vi "Apply_RF.vi"(0 "I- index":dbl, 4 "I+ index":dbl, 5 "RF Proportional to intensity":bool, 6 "RF Target Position":i32, 7 "RF indicator":bool, 8 "RF Power":dbl, 9 "rho0":dbl[](array[numeric]), 10 "rho-":dbl[](array[numeric]), 11 "rho+":dbl[](array[numeric])) -> (1 "rho- out":dbl[](array[numeric]), 2 "rho0 out":dbl[](array[numeric]), 3 "rho+ out":dbl[](array[numeric]))   [LabVIEW 2018]
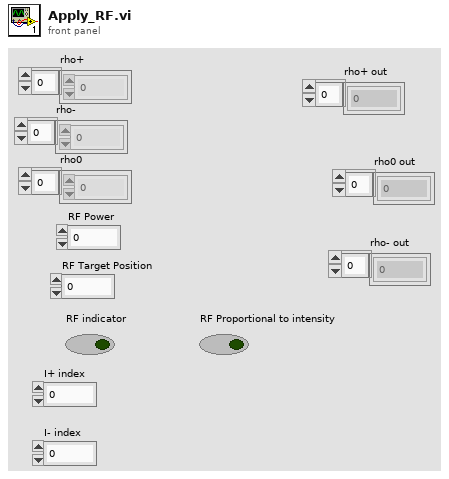
[diagram p1: front panel]
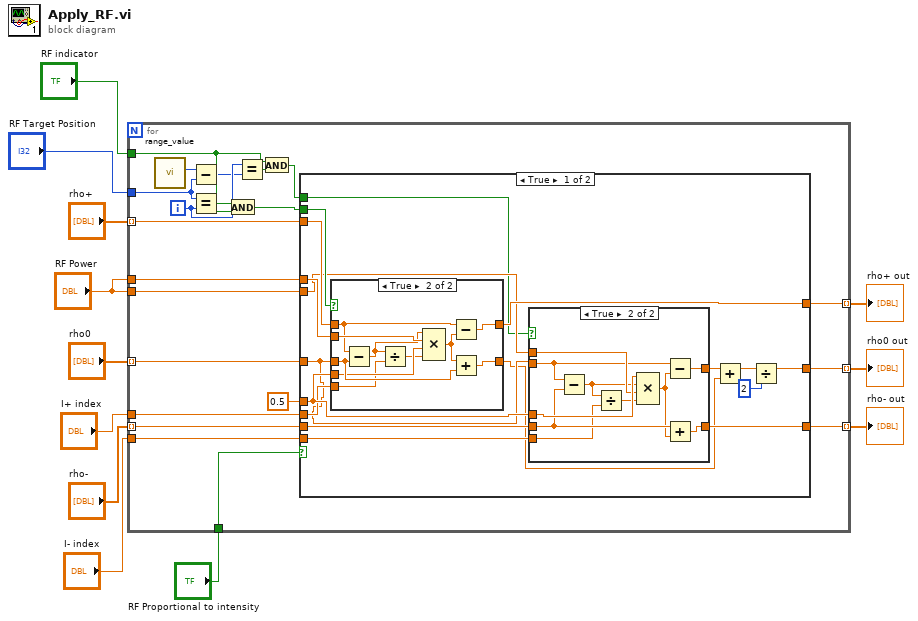
[diagram p0: block diagram]
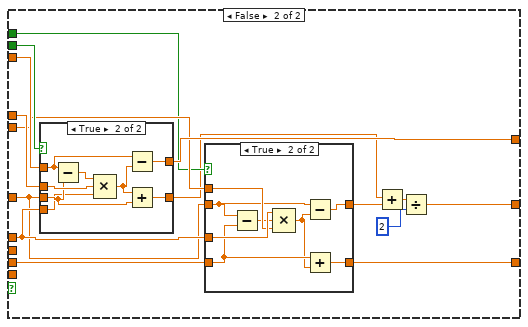
[diagram p4: hidden frame]
diagram:
  n1 = for {
    tunnel: "rho+" -> [w33] mode=indexing
    tunnel: "rho0" -> [w25] mode=indexing
    tunnel: "rho-" -> [w26] mode=indexing
    tunnel: "RF Power" -> [w30]
    tunnel: "RF Target Position" -> [w21]
    tunnel: [w31] -> w8 mode=indexing
    tunnel: [w23] -> w7 mode=indexing
    tunnel: [w28] -> w6 mode=indexing
    tunnel: "RF indicator" -> [w18]
    tunnel: "RF Power" -> [w27]
    tunnel: "I+ index" -> [w16]
    tunnel: "I- index" -> [w15]
    tunnel: "RF Proportional to intensity" -> [w14]
    i -> [w20]
    n2 = call "range_value.vi"() -> ("NumBins"=w22:i32)  [unwired: 10 in, 1 out]
    n3 = Subtract(x=w22, y=w21) -> (x-y=w13:i32)
    n4 = Equal?(x=w21, y=w20) -> (x = y?=w32:bool)
    n5 = And(x=w32, y=w18) -> (x .and. y?=w29:bool)
    n6 = Equal?(x=w20, y=w13) -> (x = y?=w19:bool)
    n7 = And(x=w18, y=w19) -> (x .and. y?=w17:bool)
    n8 = case shown="True" w14 {
      tunnel: w33 -> [w50 w89]
      tunnel: [w49 w88] -> w31
      tunnel: w30 -> [w48 w87]
      tunnel: w29 -> [w47 w86]
      tunnel: [w46 w85] -> w28
      tunnel: w27 -> [w45 w84]
      tunnel: w26 -> [w44 w83]
      tunnel: w25 -> [w38 w79]
      tunnel: 0.5 -> [w43 w82]
      tunnel: [w35 w77] -> w23
      tunnel: w17 -> [w41 w80]
      tunnel: w16 -> [w40 _]
      tunnel: w15 -> [w39 _]
      frame True {
        n9 = case shown="True" w47 {
          tunnel: w50 -> [w64 w72]
          tunnel: w38 -> [w63 w69]
          tunnel: [w64 w71] -> w49
          tunnel: [w63 w70] -> w36
          tunnel: w48 -> [_ w74]
          tunnel: w43 -> [_ w68]
          tunnel: w40 -> [_ w66]
          frame False {
          }
          frame True {
            n10 = Subtract(x=w72, y=w69) -> (x-y=w65:dbl)
            n11 = Divide(x=w65, y=w66) -> (x/y=w67:dbl)
            n12 = Compound Arithmetic op=MULTIPLY(w65, w74, w68, w67) -> (w73:dbl)
            n13 = Subtract(x=w72, y=w73) -> (x-y=w71:dbl)
            n14 = Add(x=w73, y=w69) -> (x+y=w70:dbl)
          }
        }
        n15 = case shown="True" w41 {
          tunnel: [w51 w62] -> w46
          tunnel: w43 -> [_ w61]
          tunnel: w45 -> [_ w60]
          tunnel: w44 -> [w51 w59]
          tunnel: w38 -> [w52 w57]
          tunnel: [w52 w56] -> w42
          tunnel: w39 -> [_ w53]
          frame False {
          }
          frame True {
            n16 = Subtract(x=w57, y=w59) -> (x-y=w54:dbl)
            n17 = Divide(x=w54, y=w53) -> (x/y=w55:dbl)
            n18 = Compound Arithmetic op=MULTIPLY(w61, w54, w60, w55) -> (w58:dbl)
            n19 = Subtract(x=w57, y=w58) -> (x-y=w56:dbl)
            n20 = Add(x=w59, y=w58) -> (x+y=w62:dbl)
          }
        }
        n21 = Add(x=w42, y=w36) -> (x+y=w37:dbl)
        n22 = Divide(x=w37, y=2) -> (x/y=w35:dbl)
      }
      frame False {
        n23 = case shown="True" w86 {
          tunnel: w89 -> [w101 w106]
          tunnel: w79 -> [w100 w103]
          tunnel: [w101 w105] -> w88
          tunnel: [w100 w104] -> w78
          tunnel: w87 -> [_ w108]
          tunnel: w82 -> [_ w102]
          frame False {
          }
          frame True {
            n24 = Subtract(x=w106, y=w103) -> (x-y=w109:dbl)
            n25 = Compound Arithmetic op=MULTIPLY(w109, w108, w102) -> (w107:dbl)
            n26 = Subtract(x=w106, y=w107) -> (x-y=w105:dbl)
            n27 = Add(x=w107, y=w103) -> (x+y=w104:dbl)
          }
        }
        n28 = case shown="True" w80 {
          tunnel: [w90 w99] -> w85
          tunnel: w82 -> [_ w98]
          tunnel: w84 -> [_ w97]
          tunnel: w83 -> [w90 w95]
          tunnel: w79 -> [w91 w93]
          tunnel: [w91 w92] -> w81
          frame False {
          }
          frame True {
            n29 = Subtract(x=w93, y=w95) -> (x-y=w96:dbl)
            n30 = Compound Arithmetic op=MULTIPLY(w98, w96, w97) -> (w94:dbl)
            n31 = Subtract(x=w93, y=w94) -> (x-y=w92:dbl)
            n32 = Add(x=w95, y=w94) -> (x+y=w99:dbl)
          }
        }
        n33 = Add(x=w78, y=w81) -> (x+y=w76:dbl)
        n34 = Divide(x=w76, y=2) -> (x/y=w77:dbl)
      }
    }
  }
  "rho+ out" <- w8
  "rho0 out" <- w7
  "rho- out" <- w6
